vi "DrawSelection.vi"(8 "error in (no error)":errorcluster, 11 "Menu in":refnum<class "Menu.lvclass">) -> (0 "error out":errorcluster, 3 "Menu out":refnum<class "Menu.lvclass">)   [LabVIEW 2019, in "RT_Game.lvlib" / "Menu.lvclass"]
uses:
  Menu.lvclass
  C:/Users/FreshBob/Dropbox/VIs/myRIO_GameConsole/RT/RT_Game/Game/Game.lvclass
  Game/Coordinate.ctl
  Menu.lvclass/Menu.ctl
  Game/Game.lvclass
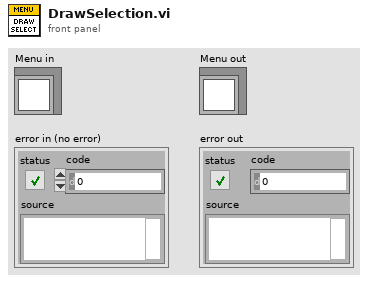
[diagram p1: front panel]
types:
  T1 = typedef "RT_Game.lvlib/Game.lvclass/Coordinate.ctl" = cluster{"x":dbl, "y":dbl}
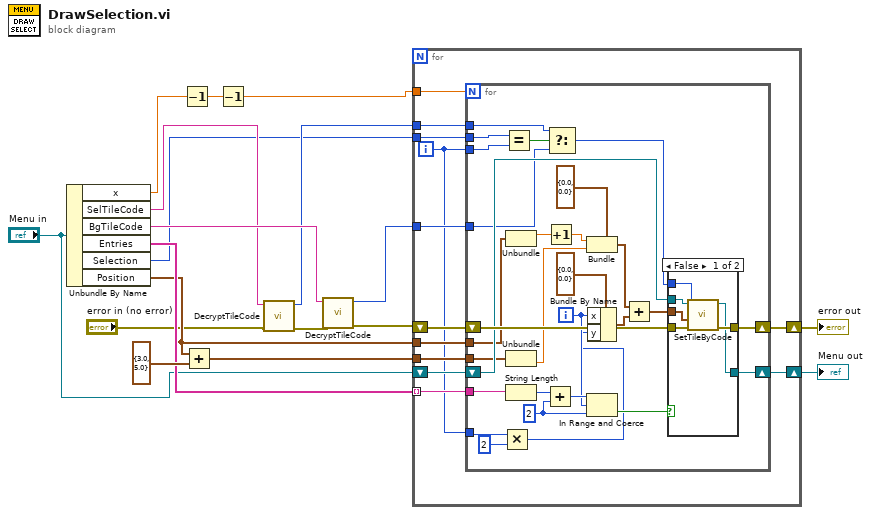
[diagram p0: block diagram]
diagram:
  n1 = Unbundle By Name("Menu in") -> ("x"=w11:dbl, "SelTileCode"=w3:string, "BgTileCode"=w7:string, "Entries"=w17:string[], "Selection"=w1:i8, "Position"=w12:T1)
  n2 = Decrement(x=w11) -> (x-1=w10:dbl)
  n3 = Add(x=w12, y=T1 {"x"=3.0, "y"=5.0}) -> (x+y=w16:T1)
  n4 = Decrement(x=w10) -> (x-1=w9:dbl)
  n5 = call "DecryptTileCode.vi"("error in (no error)"="error in (no error)", "TileCode"=w3) -> ("error out"=w4:errorcluster, "TileNumber"=w2:u16)  [unwired: 7 in, 1 out]
  n6 = call "DecryptTileCode.vi"("error in (no error)"=w4, "TileCode"=w7) -> ("error out"=w8:errorcluster, "TileNumber"=w6:u16)  [unwired: 7 in, 1 out]
  n7 = for {
    tunnel: w17 -> [w24] mode=indexing
    tunnel: w6 -> [w22]
    tunnel: w1 -> [w23]
    tunnel: w16 -> [w26]
    shift-right: [w29] -> w15
    shift-left: w8 -> [w30]
    shift-right: [w27] -> w13
    shift-left: "Menu in" -> [w28]
    tunnel: w12 -> [w25]
    tunnel: w2 -> [w21]
    tunnel: w9 -> [w20]
    i -> [w19]
    n8 = for {
      N: w20 -> [_]
      tunnel: w26 -> [w54]
      tunnel: w25 -> [w52]
      tunnel: w24 -> [w45]
      tunnel: w23 -> [w41]
      tunnel: w22 -> [w31]
      tunnel: w21 -> [w38]
      shift-right: [w58] -> w29
      shift-left: w30 -> [w59]
      shift-right: [w56] -> w27
      shift-left: w28 -> [w57]
      tunnel: w19 -> [w35]
      tunnel: w19 -> [w34]
      i -> [w36]
      w46 = 2 ("lower limit")
      n9 = Multiply(x=w34, y=2) -> (x*y=w32:i32)
      n10 = Equal?(x=w41, y=w35) -> (x = y?=w39:bool)
      n11 = Unbundle(w52) -> ("x"=w51:dbl)  [unwired: 1 out]
      n12 = Unbundle(w54) -> ("y"=w53:dbl)  [unwired: 1 out]
      n13 = String Length(string=w45) -> (length=w44:i32)
      n14 = Add(x=w44, y=w46) -> (x+y=w40:i32)
      n15 = Increment(x=w51) -> (x+1=w50:dbl)
      n16 = Select(t=w38, s=w39, f=w31) -> (s? t:f=w37:u16)
      n17 = Bundle(cluster=T1 {"x"=0.0, "y"=0.0} ("y"), "x"=w50, "y"=w53) -> (w49:T1)
      n18 = In Range and Coerce(upper limit=w40, x=w36, lower limit=w46) -> (In Range?=w43:bool)  [unwired: 1 out]
      n19 = Bundle By Name(cluster=T1 {"x"=0.0, "y"=0.0} ("y"), "x"=w36, "y"=w32) -> (w47:T1)
      n20 = Add(x=w49, y=w47) -> (x+y=w42:T1)
      n21 = case shown="False" w43 {
        tunnel: w59 -> [w65 w66]
        tunnel: [w64 w66] -> w58
        tunnel: w57 -> [w63 w67]
        tunnel: [w62 w67] -> w56
        tunnel: w42 -> [w61 _]
        tunnel: w37 -> [w60 _]
        frame False {
          n22 = call "SetTileByCode.vi"("error in (no error)"=w65, "Coordinates"=w61, "TileNumber"=w60, "Game in"=w63) -> ("error out"=w64:errorcluster, "Game out"=w62:refnum<class "Menu.lvclass">)  [unwired: 6 in]
        }
        frame True {
        }
      }
    }
  }
  "error out" <- w15
  "Menu out" <- w13
